vi "Test Bench.vi"() -> ()   [LabVIEW 2017, in "Test Bench.lvlib"]
uses:
  Test Bench/Test Bench.lvlib
  <vilib>/userdefined/High Color/nirio_resource_hc.ctl
  Test Bench/Action States.ctl
  Test Bench/Scan Engine States.ctl
  Test Bench/Scan Engine Variables.ctl
  <instrlib>/_niInstr/FIFO Register Bus/v1/Host/niInstr FIFO Register Bus v1 Host.lvclass
  <instrlib>/_niInstr/Instruction Framework/v1/Host/Instruction Framework Context/niInstr Instruction Framework Context v1 Host.lvclass
panel:
  in  "Offset":dbl(slide) min=-10.0 max=10.0 step=0.001 scale=-10.0..10.0 scale format="%#.3g"
  out "Input":bool[](array[boolean])
  in  "Output?":bool[](array[boolean])
  in  "Direction":bool[](array[boolean])
  in  "Resource Name":T1
  in  "Stop":bool
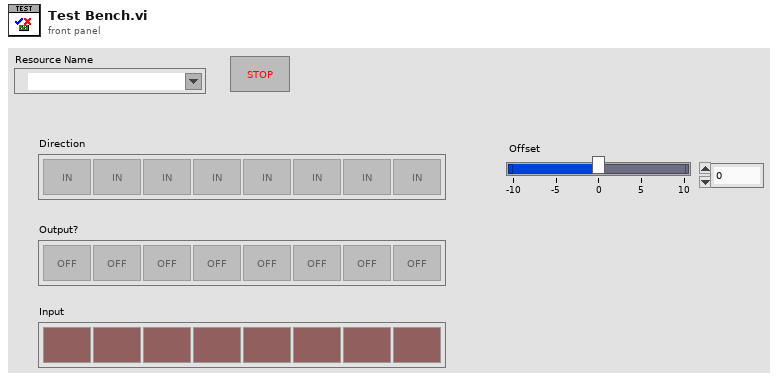
[diagram p1: front panel]
types:
  T1 = typedef "nirio_resource_hc.ctl" = tag
  T2 = typedef "Test Bench.lvlib/Scan Engine Variables.ctl" = cluster{"FPGA VI Reference":refnum<k20>, "Instruction Target":refnum<class "niInstr FIFO Register Bus v1 Host.lvclass">, "Contexts":cluster{"Digital IO":refnum<class "niInstr Instruction Framework Context v1 Host.lvclass">, "Analog Output":refnum<class "niInstr Instruction Framework Context v1 Host.lvclass">}}
  T3 = typedef "Test Bench.lvlib/Scan Engine States.ctl" = enum16{"Init", "Wait for Action", "Exit"}
  T4 = typedef "Test Bench.lvlib/Action States.ctl" = enum16{"Reset", "Update DIO Registers", "Read DI States", "Update AO Registers", "Exit"}
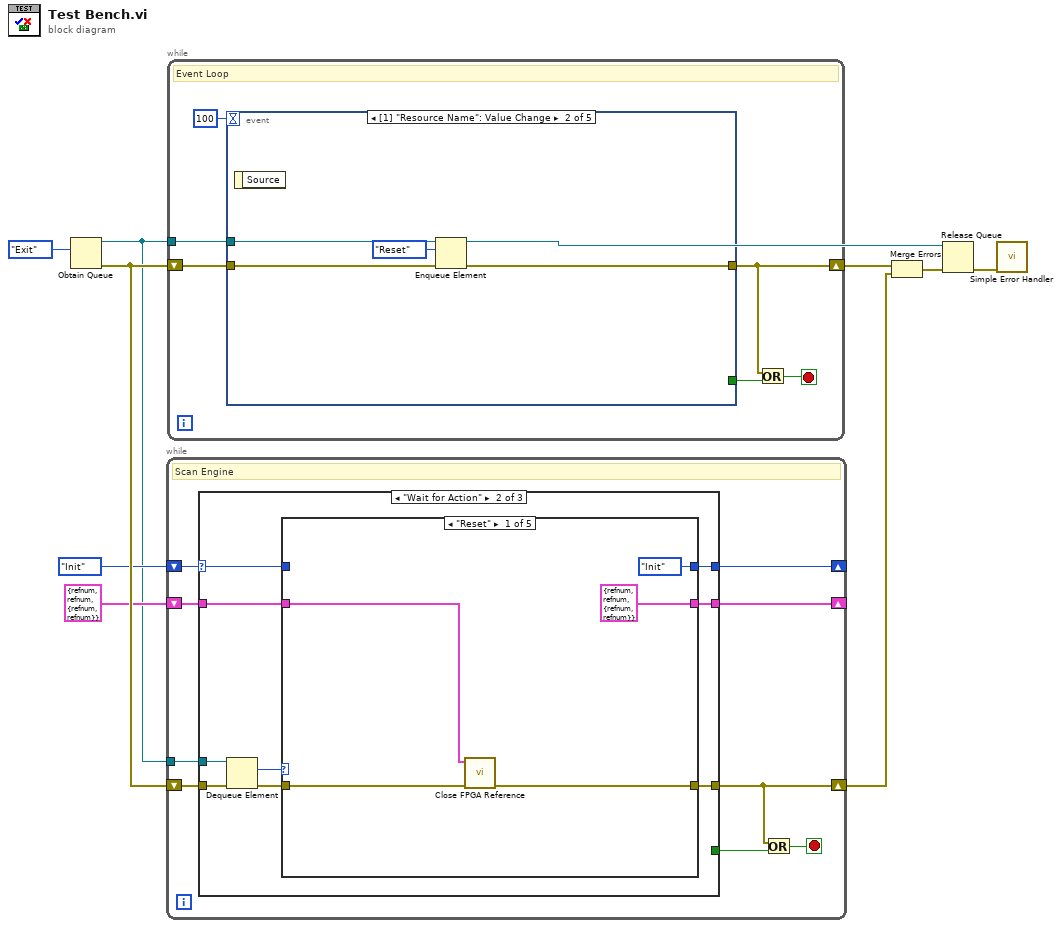
[diagram p0: block diagram]
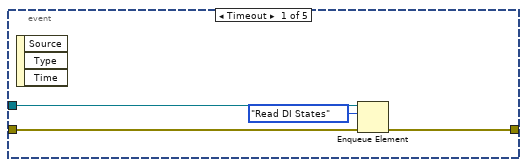
[diagram p2: hidden frame]
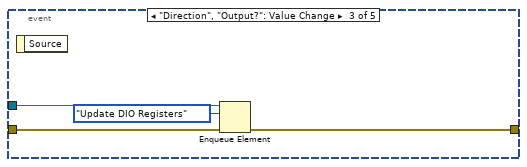
[diagram p3: hidden frame]
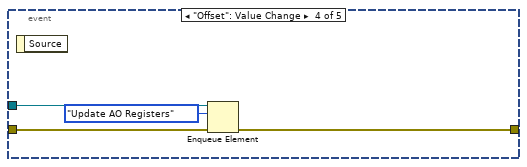
[diagram p4: hidden frame]
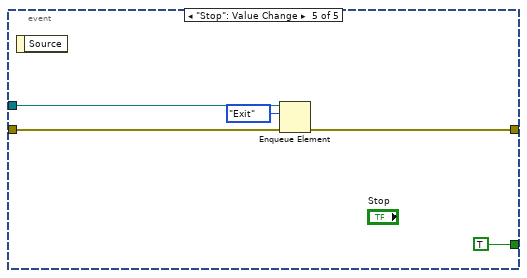
[diagram p5: hidden frame]
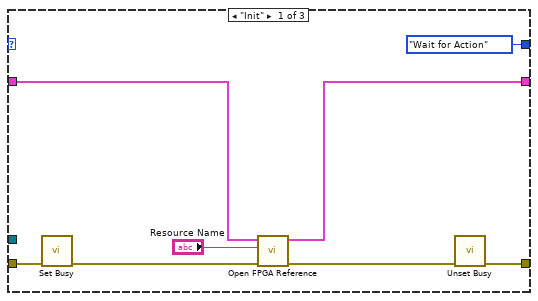
[diagram p6: hidden frame]
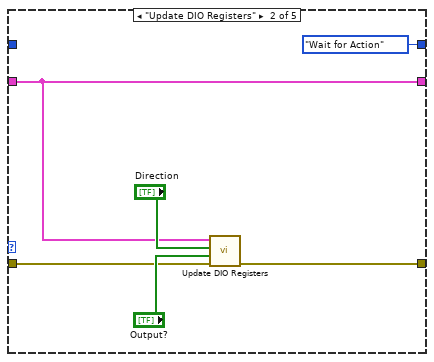
[diagram p7: hidden frame]
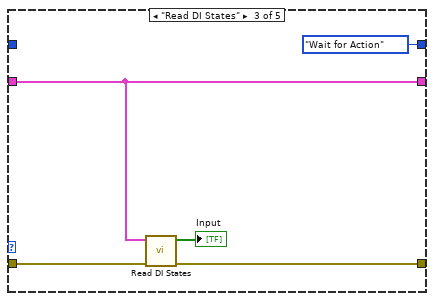
[diagram p8: hidden frame]
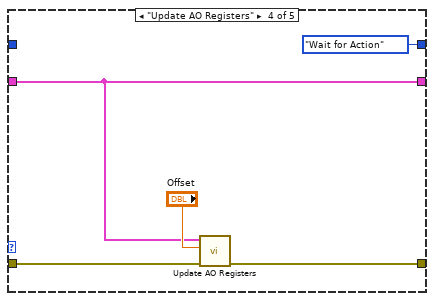
[diagram p9: hidden frame]
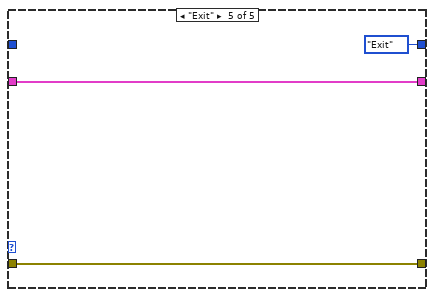
[diagram p10: hidden frame]
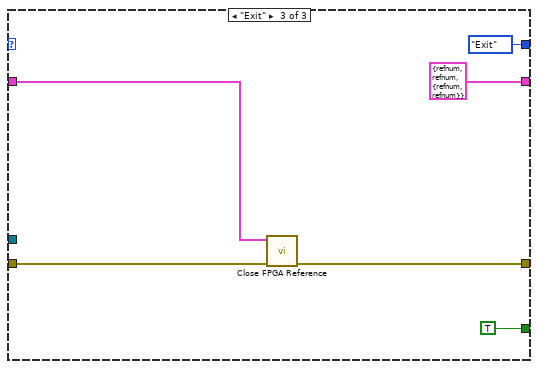
[diagram p11: hidden frame]
diagram:
  n1 = Obtain Queue(element data type=Action_States."Exit") -> (queue out=w2:refnum<queue>, error out=w8:errorcluster)  [unwired: 4 in, 1 out]
  n2 = while {
    tunnel: w2 -> [w10]
    shift-right: [w14] -> _
    shift-left: Scan_Engine_States."Init" -> [w17]
    shift-right: [w15] -> _
    shift-left: T2 {"FPGA VI Reference"=refnum, "Instruction Target"=refnum, "Contexts"={"Digital IO"=refnum, "Analog Output"=refnum}} -> [w16]
    shift-right: [w13] -> w4
    shift-left: w8 -> [w11]
    stop <- w18 stop-if-true
    # "Scan Engine"
    n3 = case shown="\"Wait for Action\"" w17 {
      selector: w17 -> [_ w31 _]
      tunnel: w16 -> [w25 w33 w62]
      tunnel: [w24 w34 T2 {"FPGA VI Reference"=refnum, "Instruction Target"=refnum, "Contexts"={"Digital IO"=refnum, "Analog Output"=refnum}}] -> w15
      tunnel: [Scan_Engine_States."Wait for Action" w32 Scan_Engine_States."Exit"] -> w14
      tunnel: w11 -> [w22 w30 w63]
      tunnel: [w19 w35 w61] -> w13
      tunnel: [_ _ TRUE] -> w12
      tunnel: w10 -> [_ w27 _]
      frame "Init" {
        n4 = call <vilib>:"Set Busy.vi"("error in (no error)"=w22) -> ("error out"=w21:errorcluster)  [unwired: 9 in, 1 out]
        n5 = call "Open FPGA Reference.vi"("error in (no error)"=w21, "Resource Name"="Resource Name", "Data in"=w25) -> ("error out"=w20:errorcluster, "Data out"=w24:T2)  [unwired: 7 in]
        n6 = call <vilib>:"Unset Busy.vi"("error in (no error)"=w20) -> ("error out"=w19:errorcluster)  [unwired: 10 in]
      }
      frame "Wait for Action" {
        n7 = Dequeue Element(queue=w27, error in (no error)=w30) -> (element=w28:T4, error out=w29:errorcluster)  [unwired: 1 in, 2 out]
        n8 = case shown="\"Reset\"" w28 {
          tunnel: w29 -> [w38 w44 w50 w54 w57]
          tunnel: [w37 w43 w49 w55 w57] -> w35
          tunnel: [T2 {"FPGA VI Reference"=refnum, "Instruction Target"=refnum, "Contexts"={"Digital IO"=refnum, "Analog Output"=refnum}} w42 w48 w52 w58] -> w34
          tunnel: w33 -> [w39 w42 w48 w52 w58]
          tunnel: [Scan_Engine_States."Init" Scan_Engine_States."Wait for Action" Scan_Engine_States."Wait for Action" Scan_Engine_States."Wait for Action" Scan_Engine_States."Exit"] -> w32
          tunnel: w31 -> [_ _ _ _ _]
          frame "Reset" {
            n9 = call "Close FPGA Reference.vi"("error in (no error)"=w38, "Data in"=w39) -> ("error out"=w37:errorcluster)  [unwired: 9 in]
          }
          frame "Update DIO Registers" {
            n10 = call "Update DIO Registers.vi"("error in (no error)"=w44, "Output?"="Output?", "Direction"="Direction", "Data"=w42) -> ("error out"=w43:errorcluster)  [unwired: 7 in]
          }
          frame "Read DI States" {
            n11 = call "Read DI States.vi"("error in (no error)"=w50, "Data in"=w48) -> ("error out"=w49:errorcluster, "States"=→"Input":bool[])  [unwired: 8 in]
          }
          frame "Update AO Registers" {
            n12 = call "Update AO Registers.vi"("error in (no error)"=w54, "Offset"="Offset", "Data in"=w52) -> ("error out"=w55:errorcluster)  [unwired: 8 in]
          }
          frame "Exit" {
          }
        }
      }
      frame "Exit" {
        n13 = call "Close FPGA Reference.vi"("error in (no error)"=w63, "Data in"=w62) -> ("error out"=w61:errorcluster)  [unwired: 9 in]
      }
    }
    n14 = Or(x=w13, y=w12) -> (x .or. y?=w18:bool)
  }
  n15 = while {
    tunnel: w2 -> [w71]
    shift-right: [w67] -> w5
    shift-left: w8 -> [w70]
    stop <- w69 stop-if-true
    # "Event Loop"
    n16 = event shown="[1] \"Resource Name\": Value Change" {
      selector: _ -> [_ _ _ _ _]
      dyn-events: _ -> [_ _ _ _ _]
      timeout: 100 -> [_ _ _ _ _]
      tunnel: w71 -> [w75 w78 w81 w86 w90]
      tunnel: w70 -> [w74 w79 w82 w87 w91]
      tunnel: [w73 w77 w83 w85 w89] -> w67
      tunnel: [_ _ _ _ TRUE] -> w68
      event Timeout {
        n17 = event-data() -> ()  [unwired: 1 in, 3 out]
        n18 = Enqueue Element(queue=w75, element=Action_States."Read DI States", error in (no error)=w74) -> (error out=w73:errorcluster)  [unwired: 1 in, 2 out]
      }
      event Value Change {
        n19 = event-data() -> ()  [unwired: 1 in, 1 out]
        n20 = Enqueue Element(queue=w78, element=Action_States."Reset", error in (no error)=w79) -> (error out=w77:errorcluster)  [unwired: 1 in, 2 out]
      }
      event "Direction", "Output?": Value Change {
        n21 = event-data() -> ()  [unwired: 1 in, 1 out]
        n22 = Enqueue Element(queue=w81, element=Action_States."Update DIO Registers", error in (no error)=w82) -> (error out=w83:errorcluster)  [unwired: 1 in, 2 out]
      }
      event "Offset": Value Change {
        n23 = event-data() -> ()  [unwired: 1 in, 1 out]
        n24 = Enqueue Element(queue=w86, element=Action_States."Update AO Registers", error in (no error)=w87) -> (error out=w85:errorcluster)  [unwired: 1 in, 2 out]
      }
      event "Stop": Value Change {
        n25 = event-data() -> ()  [unwired: 1 in, 1 out]
        n26 = Enqueue Element(queue=w90, element=Action_States."Exit", error in (no error)=w91) -> (error out=w89:errorcluster)  [unwired: 1 in, 2 out]
      }
    }
    n27 = Or(x=w67, y=w68) -> (x .or. y?=w69:bool)
  }
  n28 = Merge Errors(w5, w4) -> (w3:errorcluster)
  n29 = Release Queue(queue=w2, error in (no error)=w3) -> (error out=w1:errorcluster)  [unwired: 1 in, 2 out]
  n30 = call <vilib>:"Simple Error Handler.vi"("error in (no error)"=w1) -> ()  [unwired: 4 in, 5 out]
